vi "Create Circle Plot.vi"(11 "Circle Descr":T1) -> (3 "Points":cluster{dbl, dbl}[](array[cluster]))   [LabVIEW 2023]
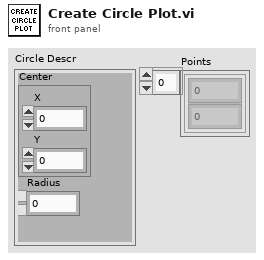
[diagram p1: front panel]
types:
  T1 = cluster{"Center":cluster{"X":sgl, "Y":sgl}, "Radius":dbl}
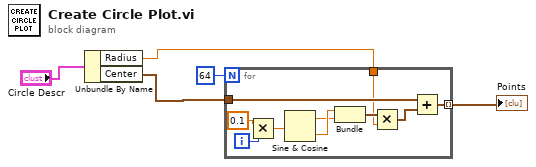
[diagram p0: block diagram]
diagram:
  n1 = Unbundle By Name("Circle Descr") -> ("Radius"=w2:dbl, "Center"=w1:cluster{"X":sgl, "Y":sgl})
  n2 = for {
    N: 64 -> [_]
    tunnel: w1 -> [w10]
    tunnel: [w9] -> w5 mode=indexing
    tunnel: w2 -> [w7]
    i -> [w15]
    n3 = Multiply(x=0.1, y=w15) -> (x*y=w11:dbl)
    n4 = Sine & Cosine(0:w11) -> (1:w12:dbl, 2:w13:dbl)
    n5 = Bundle(w13, w12) -> (w8:cluster{dbl, dbl})  [unwired: 1 in]
    n6 = Multiply(x=w8, y=w7) -> (x*y=w6:cluster{dbl, dbl})
    n7 = Add(x=w10, y=w6) -> (x+y=w9:cluster{dbl, dbl})
  }
  "Points" <- w5
